vi "Hardware Out - NI 9269-1 (Analog Output).vi"(11 "FPGA Ref":T1) -> ()   [LabVIEW 2015, in "ECS-RT.lvlib"]
uses:
  ECS-RT.lvlib
  Typedefs/FPGA Refs/Generic FPGA Ref.ctl
  <vilib>/Utility/error.llb/Error Cluster From Error Code.vi
  <vilib>/rvi/errors/niLvFpgaAdjustHostInterfaceError.vi
  <vilib>/rvi/interface/nirviReadWriteControl/nirviReadWriteControl.xnode
  <vilib>/rvi/interface/Simulation/niFpgaSimulationCallBeginRW.vi
  NiFpgaLv.dll
  ECS-Shared.lvlib
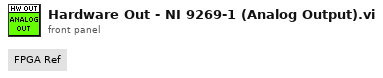
[diagram p1: front panel]
types:
  T1 = typedef "ECS-Shared.lvlib/Generic FPGA Ref.ctl" = refnum<k20>
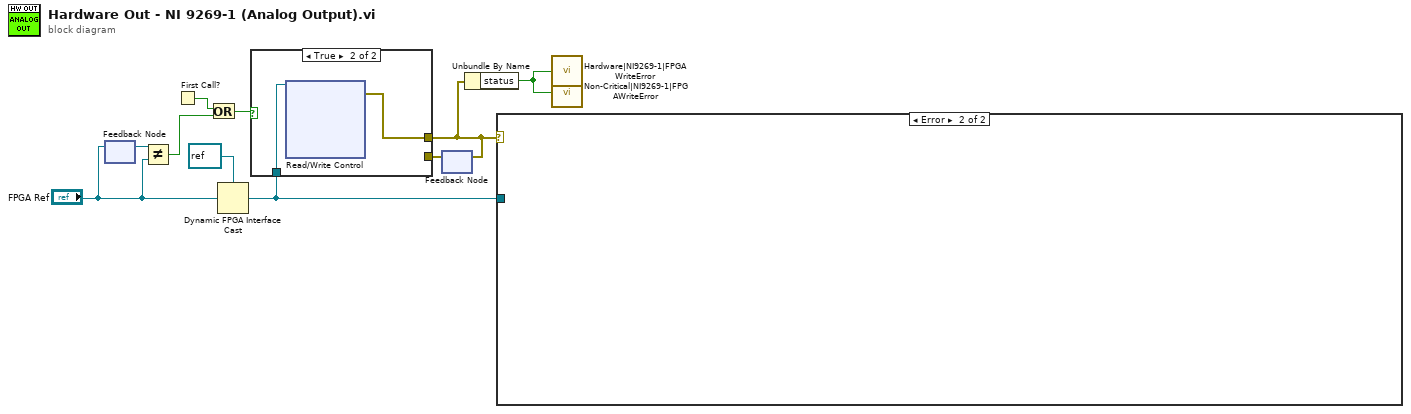
[diagram p0: block diagram]
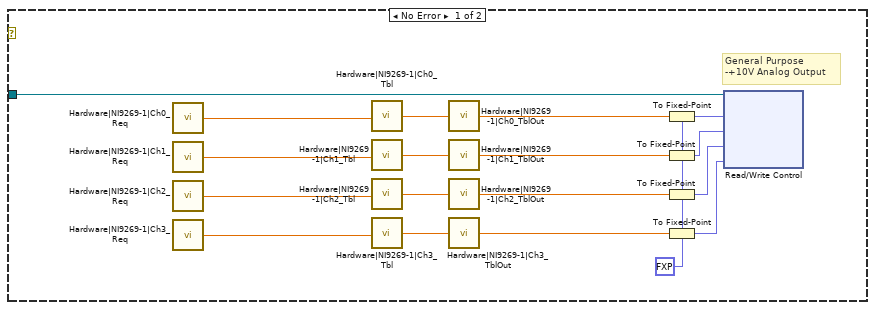
[diagram p3: hidden frame]
diagram:
  n1 = feedback #1() -> (w7:T1)  [unwired: 1 in]
  n2 = feedback-in #1("FPGA Ref") -> ()
  n3 = Not Equal?(x=w7, y="FPGA Ref") -> (x != y?=w6:bool)
  n4 = First Call?() -> (First Call?: T/F=w8:bool)
  n5 = Or(x=w8, y=w6) -> (x .or. y?=w9:bool)
  n6 = Dynamic FPGA Interface Cast(Session In=refnum<k20> refnum ("NI 9269"), Type="FPGA Ref") -> (Session Out=w5:refnum<k20>)
  n7 = feedback #2() -> (w10:errorcluster)  [unwired: 1 in]
  n8 = case shown="True" w9 {
    tunnel: [w11 w13] -> w2
    tunnel: w10 -> [w11 _]
    tunnel: w5 -> [_ w12]
    frame False {
    }
    frame True {
      n9 = xnode "Read/Write Control"("FPGA VI Reference In"=w12) -> ("error out"=w13:errorcluster)  [unwired: 5 in, 1 out]
    }
  }
  n10 = feedback-in #2(w2) -> ()
  n11 = Unbundle By Name(w2) -> ("status"=w1:bool)
  n12 = case shown="Error" w2 {
    tunnel: w5 -> [w14 _]
    frame No Error {
      w17 = fxp<+/-,20,5> 0.0 ("9269.AO0")
      # "General Purpose\n-+10V Analog Output"
      n13 = call "Hardware|NI9269-1|Ch0_Req"() -> ("Value"=w27:sgl)
      n14 = call "Hardware|NI9269-1|Ch1_Req"() -> ("Value"=w26:sgl)
      n15 = call "Hardware|NI9269-1|Ch2_Req"() -> ("Value"=w25:sgl)
      n16 = call "Hardware|NI9269-1|Ch3_Req"() -> ("Value"=w24:sgl)
      n17 = call "Hardware|NI9269-1|Ch0_Tbl"("X Index"=w27) -> ("Y"=w20:sgl)
      n18 = call "Hardware|NI9269-1|Ch1_Tbl"("X Index"=w26) -> ("Y"=w21:sgl)
      n19 = call "Hardware|NI9269-1|Ch2_Tbl"("X Index"=w25) -> ("Y"=w22:sgl)
      n20 = call "Hardware|NI9269-1|Ch3_Tbl"("X Index"=w24) -> ("Y"=w23:sgl)
      n21 = call "Hardware|NI9269-1|Ch0_TblOut"("Value"=w20) -> ()
      n22 = call "Hardware|NI9269-1|Ch1_TblOut"("Value"=w21) -> ()
      n23 = call "Hardware|NI9269-1|Ch2_TblOut"("Value"=w22) -> ()
      n24 = call "Hardware|NI9269-1|Ch3_TblOut"("Value"=w23) -> ()
      n25 = To Fixed-Point(fixed-point type=w17, number=w20) -> (fixed-point=w19:fxp<+/-,20,5>)
      n26 = To Fixed-Point(fixed-point type=w17, number=w21) -> (fixed-point=w18:fxp<+/-,20,5>)
      n27 = To Fixed-Point(fixed-point type=w17, number=w22) -> (fixed-point=w16:fxp<+/-,20,5>)
      n28 = To Fixed-Point(fixed-point type=w17, number=w23) -> (fixed-point=w15:fxp<+/-,20,5>)
      n29 = xnode "Read/Write Control"("FPGA VI Reference In"=w14, "9269-1.AO0"=w19, "9269-1.AO1"=w18, "9269-1.AO2"=w16, "9269-1.AO3"=w15) -> ()  [unwired: 1 in, 2 out]
    }
    frame Error {
    }
  }
  n30 = call "Hardware|NI9269-1|FPGAWriteError"("Value"=w1) -> ()
  n31 = call "Non-Critical|NI9269-1|FPGAWriteError"("Fault"=w1) -> ()  [unwired: 2 in]
